vi "Return Round-Trip Message.vi"(8 "error in (no error)":errorcluster, 11 "RoundTripMessage In":refnum<class "RoundTripMessage.lvclass">) -> (0 "error out":errorcluster)   [LabVIEW 2019, in "RoundTripMessage.lvclass"]
uses:
  <vilib>/gpm_packages/@cs/actor-framework-messages/Source/RoundTripMessage/RoundTripMessage.lvclass
  C:/Program Files/National Instruments/LabVIEW 2019/vi.lib/ActorFramework/Message/Message.lvclass
  <vilib>/gpm_packages/@cs/actor-framework-messages/Source/RoundTripMessage/RoundTripMessage.lvclass/RoundTripMessage.ctl
  <vilib>/ActorFramework/Message Enqueuer/Message Enqueuer.lvclass/Message Enqueuer.ctl
  <vilib>/ActorFramework/Message Priority Queue/Priority Enqueue.vi
  <vilib>/ActorFramework/Message Enqueuer/Message Enqueuer.lvclass
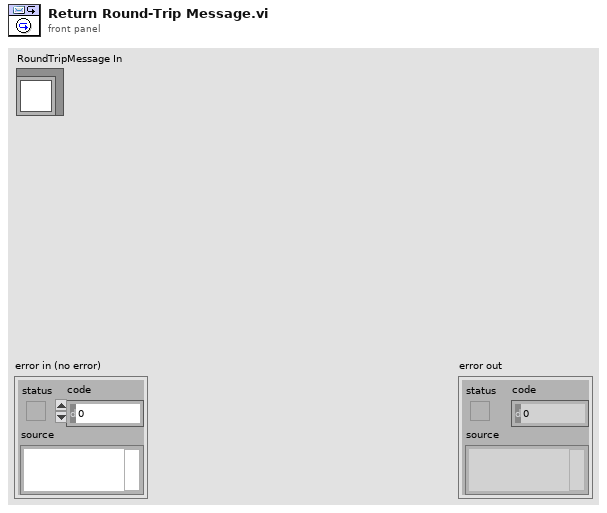
[diagram p1: front panel]
types:
  T1 = typedef "Actor Framework.lvlib/Message Enqueuer.lvclass/Message Priority.ctl" = enum16{"Low", "Normal", "High"}
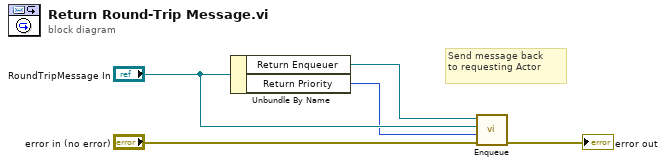
[diagram p0: block diagram]
diagram:
  # "Send message back\nto requesting Actor"
  n1 = Unbundle By Name("RoundTripMessage In") -> ("Return Enqueuer"=w3:refnum<class "Message Enqueuer.lvclass">, "Return Priority"=w1:T1)
  n2 = call <vilib>:"Enqueue.vi"("error in (no error)"="error in (no error)", "Message Priority (Normal)"=w1, "Message"="RoundTripMessage In", "Message Enqueuer in"=w3) -> ("error out"=→"error out":errorcluster)  [unwired: 6 in, 1 out]
